vi "uActor_Send_Stop.vi"(8 "error in (no error)":errorcluster, 11 "uActor Transport":refnum<class "uTransport_uActor.lvclass">) -> (0 "error out":errorcluster)   [LabVIEW 2021, in "uFramework.lvlib" / "uActor.lvclass"]
doc: "Send a STOP message to the actor even on error-in."
uses:
  uActor.lvclass
  uTransport_uActor/uTransport_uActor.lvclass
  uMsg/uMsg.lvclass/uMsg.ctl
  uTransport_uActor/uTransport_uActor.lvclass/uTransport_uActor.ctl
  uActor_SendMsg.vi
  uMsg/uMsg Create.vi
  uTransport_uActor/uTransport_uActor_SendMsg.vi
  uMsg/uMsg Update Timestamp.vi
  Bin/uData.lvlibp/uData.lvclass
  uTransport/uTransport.lvclass
  uMsg/uMsg.lvclass
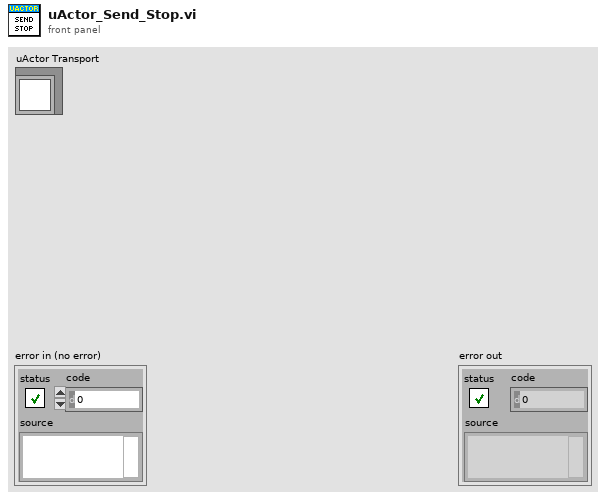
[diagram p1: front panel]
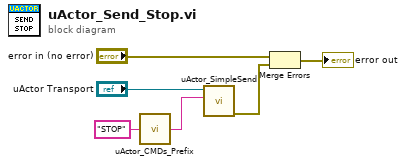
[diagram p0: block diagram]
diagram:
  n1 = call "uActor_CMDs_Prefix.vi"("uActor CMD"="STOP") -> ("Reserved CMD"=w1:string)
  n2 = call "uActor_SimpleSend.vi"("Msg"=w1, "uActor Transport"="uActor Transport") -> ("error out"=w6:errorcluster)  [unwired: 9 in]
  n3 = Merge Errors("error in (no error)", w6) -> (→"error out":errorcluster)
